vi "Get or Init IC Class Array.vi"(5 "type check? (T)":bool=TRUE, 7 "target IC":refnum<class "NI_IC.lvclass">, 8 "error in (no error)":errorcluster, 9 "index":i32, 10 "# of IC":i32, 11 "PDE in":refnum<class "NI_PDE.lvclass">) -> (0 "error out":errorcluster, 1 "IC out":refnum<class "NI_IC.lvclass">, 2 "IC Array":refnum<class "NI_IC.lvclass">[](array[class]), 3 "PDE out":refnum<class "NI_PDE.lvclass">)   [LabVIEW 2017, in "NI_PDE.lvlib" / "NI_PDE.lvclass"]
uses:
  <vilib>/gmath/pde.llb/PDEClass/NI_PDE.lvclass
  <vilib>/gmath/pde.llb/ICClass/NI_IC.lvclass
  <vilib>/gmath/pde.llb/ICClass/Class Type.ctl
  <vilib>/gmath/pde.llb/Common/PDE_Error.ctl
  <vilib>/gmath/NI_PDE.lvlib
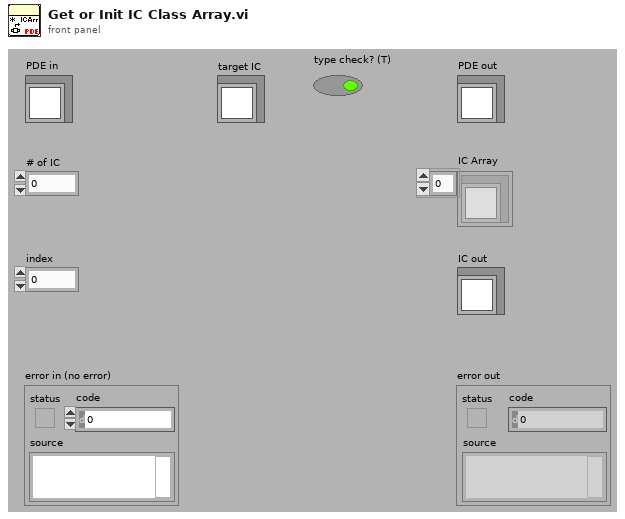
[diagram p1: front panel]
types:
  T1 = typedef "NI_PDE.lvlib/PDE_Error.ctl" = enum16{"No Error", "k is zero", "End point <= start point", "# of time steps < 2", "# of spatial points < 3", "# of grid < 1 for FEM", "# of boundary < 3 for FEM", "Incompatible RHS size", "Incompatible BC size", "Incompatible IC size", "PDE class conflict", "RHS class conflict", "Domain class conflict", "BC class conflict", "IC class conflict"}
  T2 = typedef "NI_PDE.lvlib/NI_IC.lvclass/Class Type.ctl" = i32
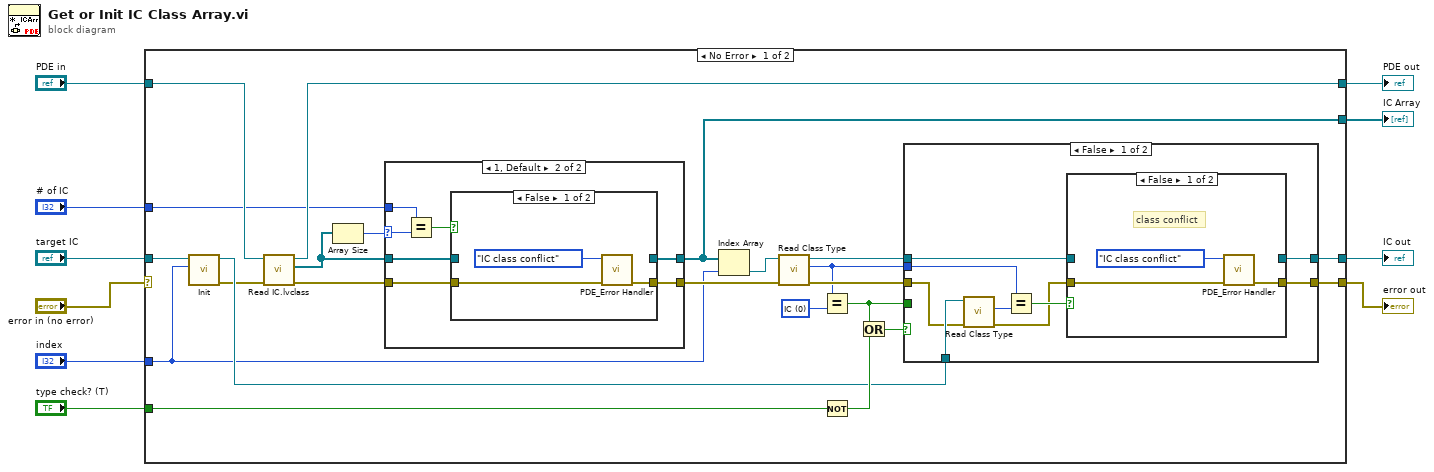
[diagram p0: block diagram]
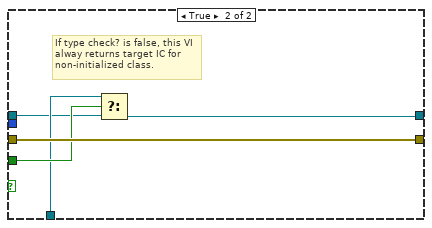
[diagram p3: hidden frame]
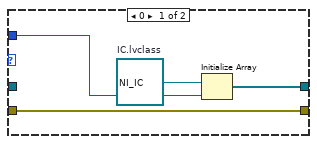
[diagram p4: hidden frame]
diagram:
  n1 = case shown="No Error" "error in (no error)" {
    selector: "error in (no error)" -> [_ w70]
    tunnel: "PDE in" -> [w33 w71]
    tunnel: [w25 w71] -> w9
    tunnel: [w24 w70] -> w8
    tunnel: "# of IC" -> [w23 _]
    tunnel: "index" -> [w11 _]
    tunnel: [w22 _] -> w5
    tunnel: [w21 w69] -> w4
    tunnel: "target IC" -> [w12 w69]
    tunnel: "type check? (T)" -> [w19 _]
    frame No Error {
      w15 = T2 0 items=["IC"=0, "IC_1D"=10, "IC_1D_Numeric"=11, "IC_1D_VIRef"=12, "IC_2D"=20, "IC_2D_Numeric"=21, "IC_2D_VIRef"=22] ("y")
      n2 = call-dynamic "Init.vi"("index"=w11, "IC"=w12) -> ("error out"=w13:errorcluster, "initialized IC"=w14:refnum<class "NI_IC.lvclass">)  [unwired: 1 in, 7 out]
      n3 = call-dynamic "Read IC.lvclass.vi"("error in (no error)"=w13, "PDE.lvclass in"=w33) -> ("error out"=w31:errorcluster, "IC.lvclass"=w30:refnum<class "NI_IC.lvclass">[], "PDE.lvclass out"=w25:refnum<class "NI_PDE.lvclass">)  [unwired: 7 out]
      n4 = Array Size(array=w30) -> (size(s)=w32:i32)
      n5 = case shown="1, Default" w32 {
        selector: w32 -> [_ w60]
        tunnel: w31 -> [w56 w63]
        tunnel: [w55 w57] -> w22
        tunnel: w30 -> [_ w58]
        tunnel: [w56 w62] -> w26
        tunnel: w23 -> [w54 w61]
        frame 0 {
          w53 = refnum<class "NI_IC.lvclass"> refnum  # IC.lvclass
          n6 = Initialize Array(w53, w54) -> (w55:refnum<class "NI_IC.lvclass">[])
        }
        frame 1, Default {
          n7 = Equal?(x=w61, y=w60) -> (x = y?=w59:bool)
          n8 = case shown="False" w59 {
            tunnel: w63 -> [w65 w67]
            tunnel: [w64 w67] -> w62
            tunnel: w58 -> [_ w68]
            tunnel: [_ w68] -> w57
            frame False {
              n9 = call <vilib>:"PDE_Error Handler.vi"("error in (no error)"=w65, "PDE error"=PDE_Error."IC class conflict") -> ("error out"=w64:errorcluster)  [unwired: 9 out]
            }
            frame True {
            }
          }
        }
      }
      n10 = Index Array(array=w22, index=w11) -> (element=w29:refnum<class "NI_IC.lvclass">)
      n11 = call-dynamic "Read Class Type.vi"("error in (no error)"=w26, "IC.lvclass in"=w29) -> ("error out"=w27:errorcluster, "IC class type"=w20:T2, "IC.lvclass out"=w28:refnum<class "NI_IC.lvclass">)  [unwired: 7 out]
      n12 = Equal?(x=w20, y=w15) -> (x = y?=w16:bool)
      n13 = Not(x=w19) -> (.not. x?=w18:bool)
      n14 = Or(x=w16, y=w18) -> (x .or. y?=w17:bool)
      n15 = case shown="False" w17 {
        tunnel: w28 -> [w42 w49]
        tunnel: w27 -> [w35 w52]
        tunnel: [w41 w52] -> w24
        tunnel: [w40 w48] -> w21
        tunnel: w20 -> [w39 _]
        tunnel: w14 -> [w37 w50]
        tunnel: w16 -> [_ w51]
        frame False {
          n16 = call-dynamic "Read Class Type.vi"("error in (no error)"=w35, "IC.lvclass in"=w37) -> ("error out"=w34:errorcluster, "IC class type"=w36:T2)  [unwired: 8 out]
          n17 = Equal?(x=w39, y=w36) -> (x = y?=w38:bool)
          n18 = case shown="False" w38 {
            tunnel: w42 -> [_ w47]
            tunnel: w34 -> [w44 w46]
            tunnel: [_ w47] -> w40
            tunnel: [w43 w46] -> w41
            frame False {
              # "class conflict"
              n19 = call <vilib>:"PDE_Error Handler.vi"("error in (no error)"=w44, "PDE error"=PDE_Error."IC class conflict") -> ("error out"=w43:errorcluster)  [unwired: 9 out]
            }
            frame True {
            }
          }
        }
        frame True {
          # "If type check? is false, this VI alway returns target IC for non-initialized class."
          n20 = Select(t=w50, s=w51, f=w49) -> (s? t:f=w48:refnum<class "NI_IC.lvclass">)
        }
      }
    }
    frame Error {
    }
  }
  "PDE out" <- w9
  "error out" <- w8
  "IC Array" <- w5
  "IC out" <- w4
